vi "ReadTests.vi"() -> ()   [LabVIEW 2014]
uses:
  TestCase/TestCase.lvclass
  <vilib>/xml/Load XML File.vi
  <vilib>/xml/NI_XML.lvlib
panel:
  out "Array":refnum<class "TestCase.lvclass">[](array[class])
  in  "path to XML document":path
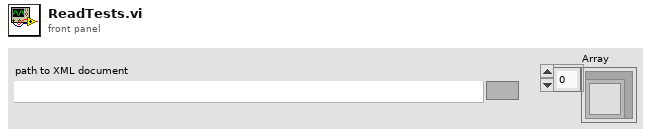
[diagram p1: front panel]
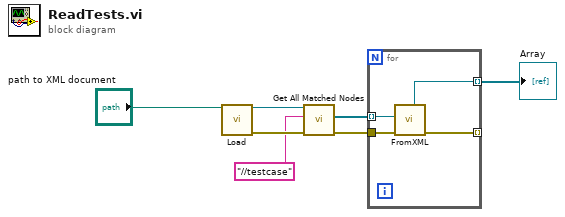
[diagram p0: block diagram]
diagram:
  n1 = call-poly <vilib>:"Load.vi"("path to XML document"="path to XML document") -> ("DOM document out"=w5:refnum<k20>, "error out"=w6:errorcluster)  [unwired: 12 in, 1 out]
  n2 = call <vilib>:"Get All Matched Nodes.vi"("error in (no error)"=w6, "XPath expression"="//testcase", "node in"=w5) -> ("error out"=w3:errorcluster, "node result array"=w2:refnum<k20>[])  [unwired: 6 in, 1 out]
  n3 = for {
    tunnel: w3 -> [w11]
    tunnel: w2 -> [w10] mode=indexing
    tunnel: [w9] -> w1 mode=indexing
    tunnel: [w8] -> _ mode=indexing
    n4 = call "FromXML.vi"("error in"=w11, "TestCase element"=w10) -> ("error out"=w8:errorcluster, "TestCase out"=w9:refnum<class "TestCase.lvclass">)  [unwired: 6 in]
  }
  "Array" <- w1
